vi "RT GV.vi"() -> ()   [LabVIEW 2015]
panel:
  in  "Th":sgl
  in  "Fre":dbl
  out "Image Disp":T1(plugin-control)
  in  "IR":cluster{"1":bool, "2":bool}
  in  "Servo Motors Control":T2={"Base"=1500, "Elbow"=1500, "Claw"=1500, "Shoulder"=1500} {"Shoulder" min=500 max=2500 scale=500.0..2500.0; "Claw" min=500 max=2500 scale=500.0..2500.0; "Elbow" min=500 max=2500 scale=500.0..2500.0; "Base" min=500 max=2500 scale=500.0..2500.0}
  in  "Control Type":bool
  in  "Image":bool
  in  "SB INIT":bool
  out "BOOL O/P":T3
  in  "Command":T4(ring)
  in  "Buttons Control":T5
  in  "Stop Button":bool
  in  "IR L - OBST AVD 3":bool
  in  "IR R - OBST AVD 2":bool
  in  "USF Combine - OBST AVD":bool
  # "Movement"
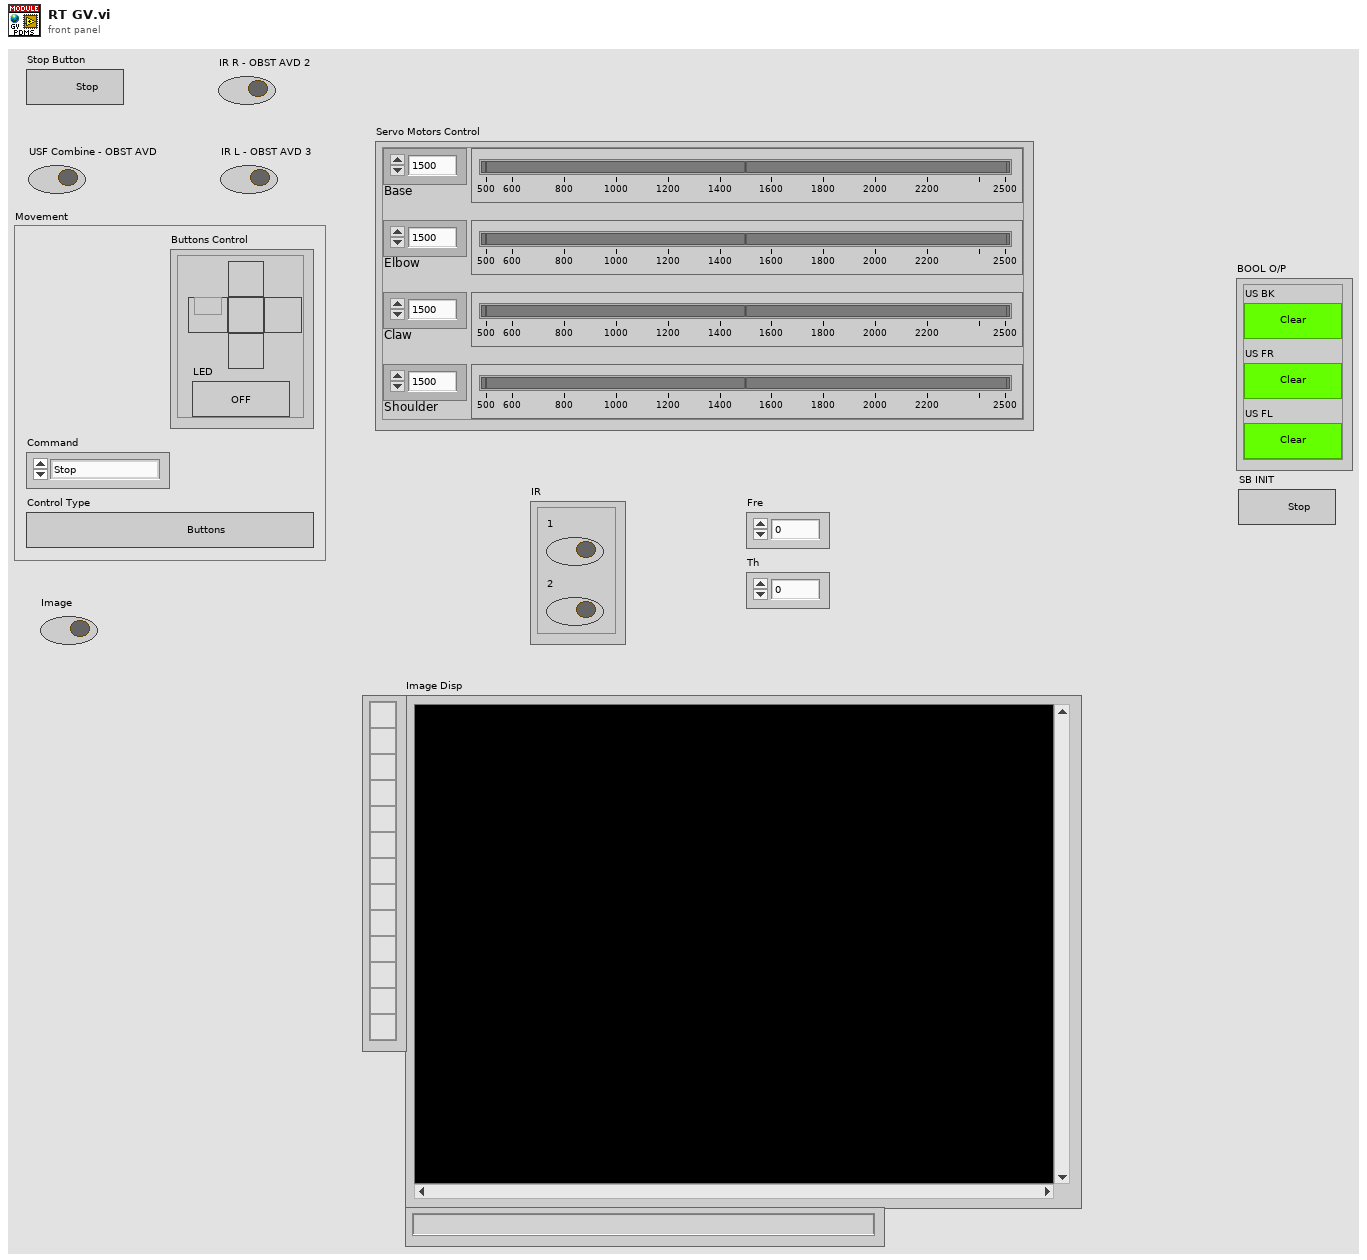
[diagram p1: front panel]
types:
  T1 = typedef "IMAQ Image.ctl" = refnum<image>
  T2 = cluster{"Base":u32, "Elbow":u32, "Claw":u32, "Shoulder":u32}
  T3 = cluster{"US BK":bool, "US FR":bool, "US FL":bool}
  T4 = enum16{"Stop", "LED", "Front", "Back", "Left", "Right"}
  T5 = cluster{"Front":bool, "Right":bool, "Back":bool, "Left":bool, "Stop":bool, "LED":bool}
diagram:
